vi "Polynom Daten speichern.vi"(6 "Aktionen":T3, 7 "Aktuelle Gasliste FT-IR":T1[](array[typedef]), 8 "Aktiv":bool[](array[boolean]), 9 "Polynome":dbl[][](array[numeric]) format="%#_18f", 10 "Einzelnes Polynom":dbl[](array[numeric]), 11 "Komponente":u16) -> (0 "Aktiv":bool[](array[boolean]), 1 "Polynome":dbl[][](array[numeric]) format="%#_18g", 2 "Namen":string[](array[string]), 3 "Polynome":T2 {"Polynom" format="%#_20f"}, 4 "Einzelnes Polynom out":dbl[](array[numeric]), 5 "einzelnes aktiv":bool)   [LabVIEW 2020, in "Linearisierung v2.lvlib"]
uses:
  Linearisierung v2.lvlib
  Aktionen Polynom Daten speichern.ctl
  Polynome.ctl
  Visualisierungs Elemente/String - Ausgabefeld.ctl
  Allgemein/allgemeine Sub-VIs.lvlib
  Seiten/Gaszuordnung AO/Gaszuordnung AO.lvlib
  Polynomkoeffizientenanzeige.ctl
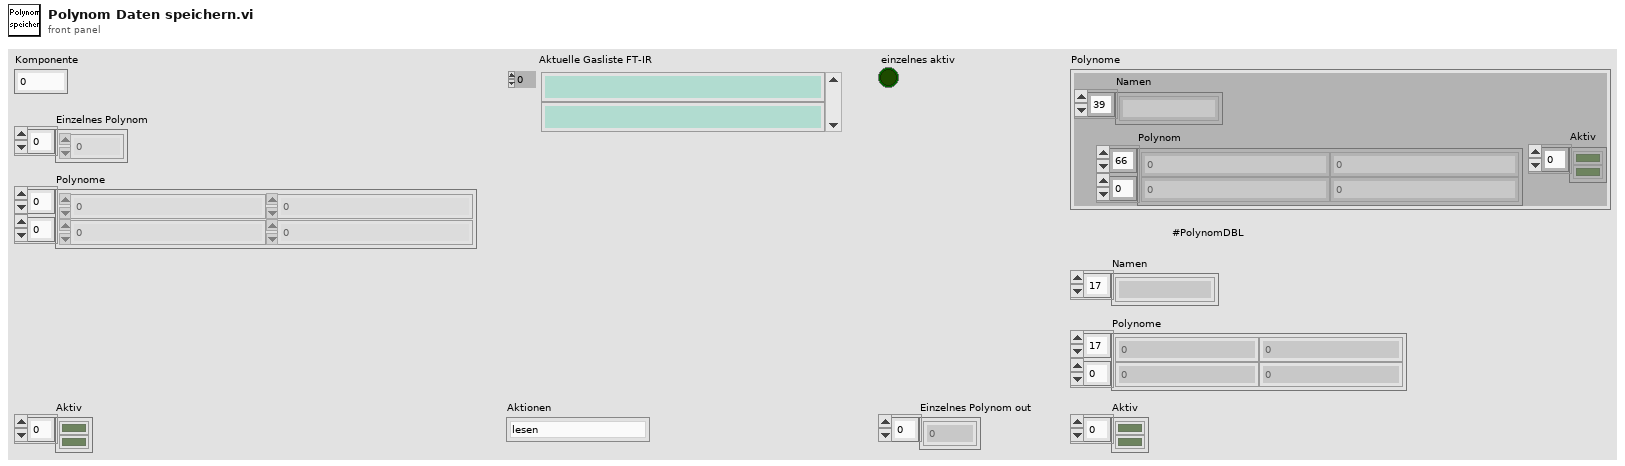
[diagram p1: front panel]
types:
  T1 = typedef "String - Ausgabefeld.ctl" = string
  T2 = typedef "Linearisierung v2.lvlib/Polynome.ctl" = cluster{"Namen":string[], "Polynom":dbl[][], "Aktiv":bool[]}
  T3 = typedef "Linearisierung v2.lvlib/Aktionen Polynom Daten speichern.ctl" = enum16{"lesen", "laden", "speichern", "schreiben", "schreiben alle", "Liste erstellen", "aktivieren", "deaktivieren", "aktiv abfragen"}
  T4 = enum16{"open", "replace", "create", "open or create", "replace or create", "replace or create with confirmation"}
  T5 = typedef "Linearisierung v2.lvlib/Polynomkoeffizientenanzeige.ctl" = cluster{"Offset":dbl, "O.1":dbl, "O. 2":dbl, "O. 3":dbl, "O. 4":dbl}
  T6 = cluster{"Namen":string[], "Polynom":dbl[][], "Aktiv":bool[]}
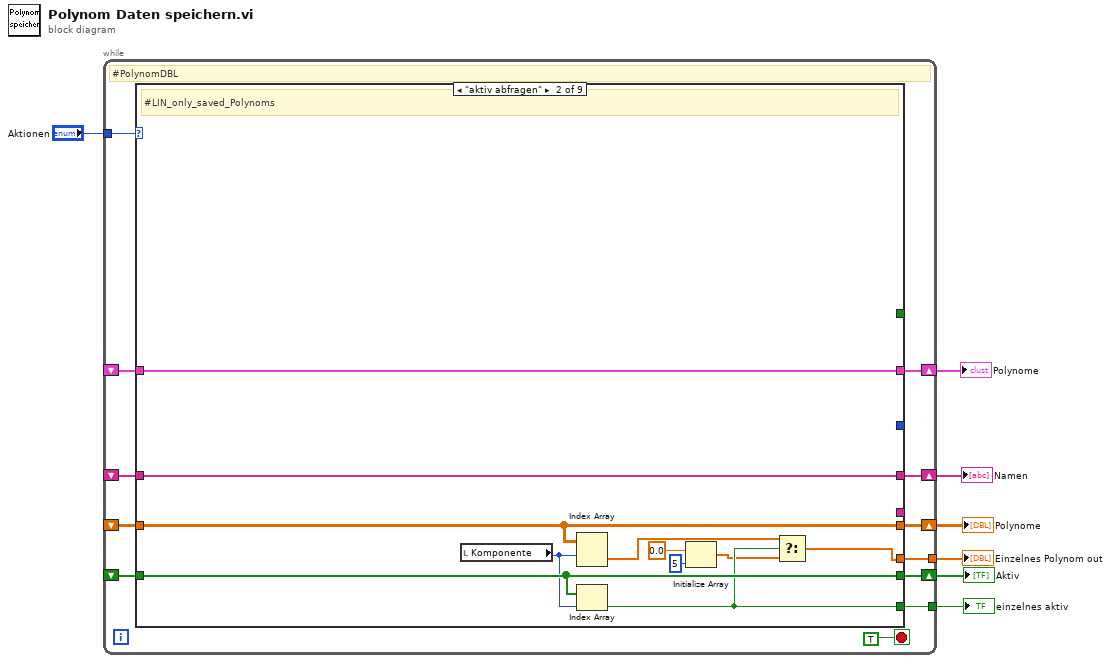
[diagram p0: block diagram]
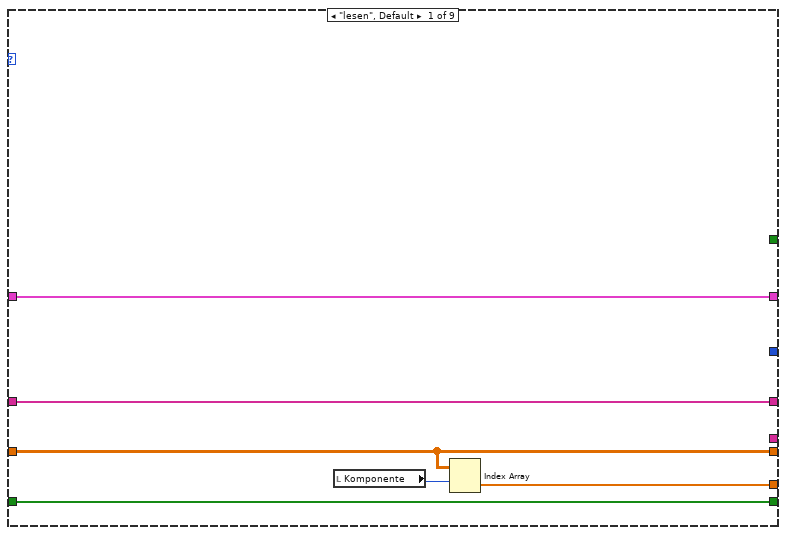
[diagram p2: hidden frame]
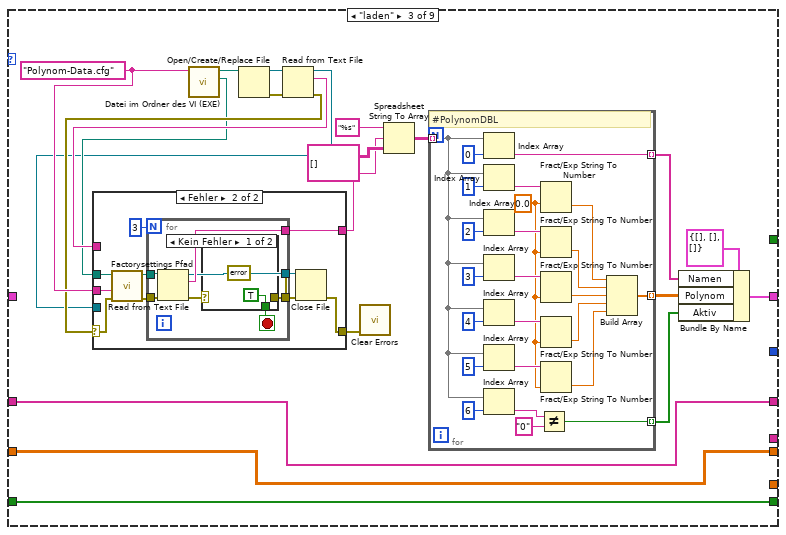
[diagram p3: hidden frame]
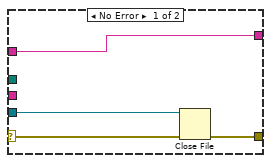
[diagram p4: hidden frame]
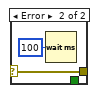
[diagram p5: hidden frame]
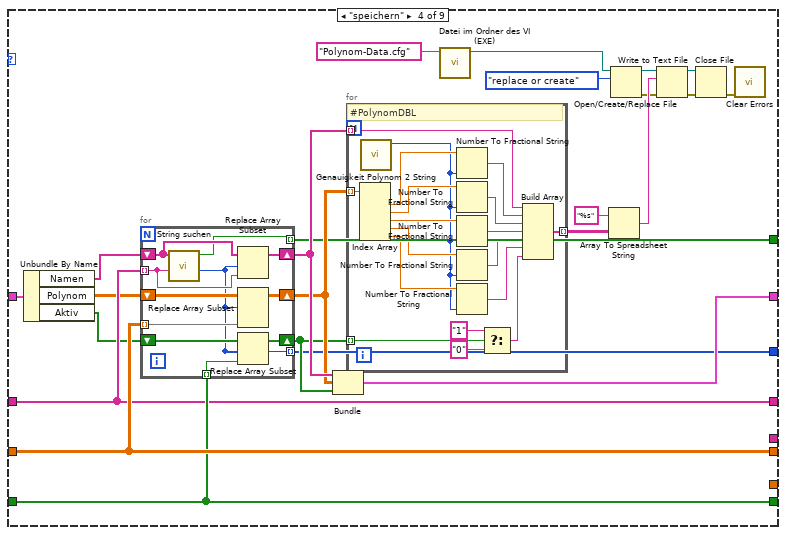
[diagram p6: hidden frame]
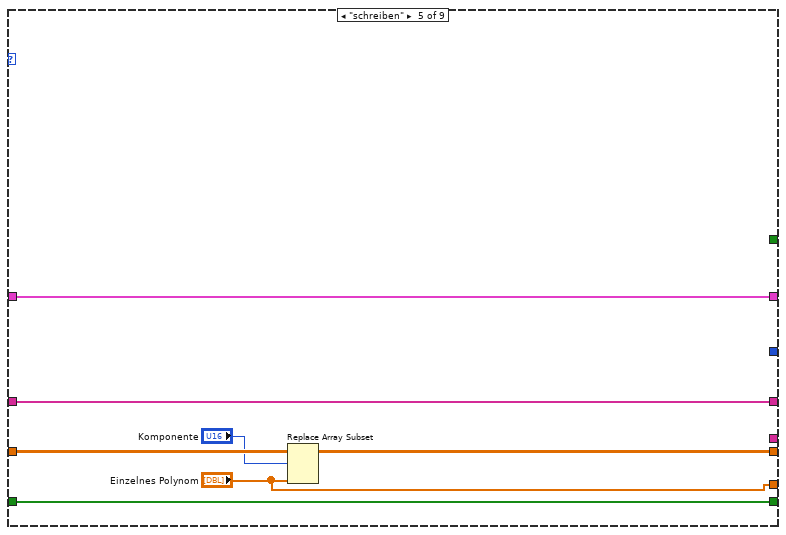
[diagram p7: hidden frame]
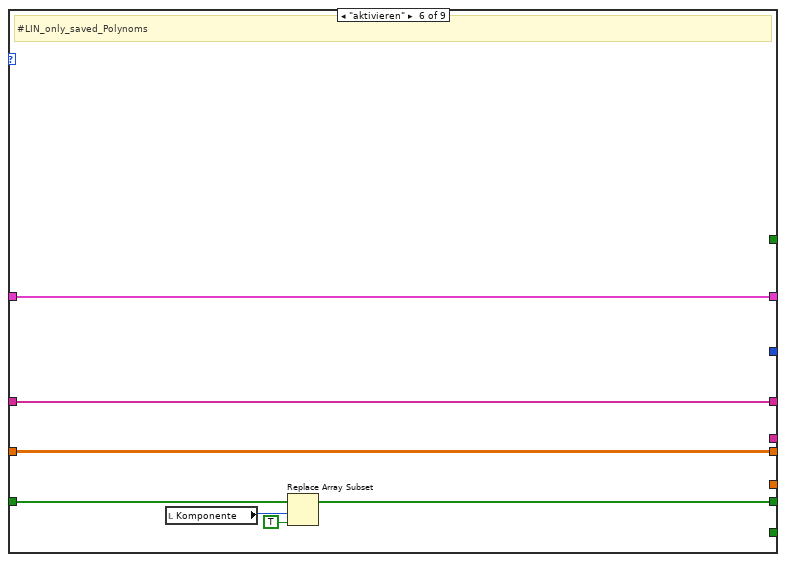
[diagram p8: hidden frame]
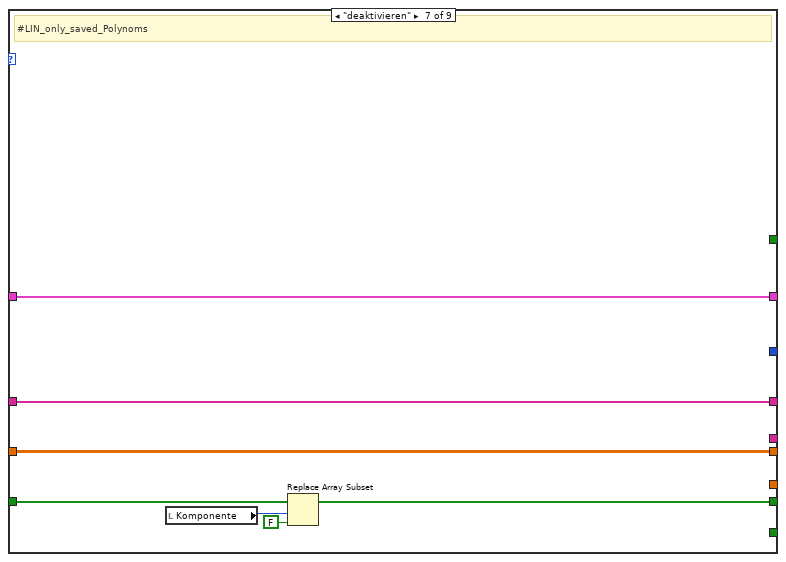
[diagram p9: hidden frame]
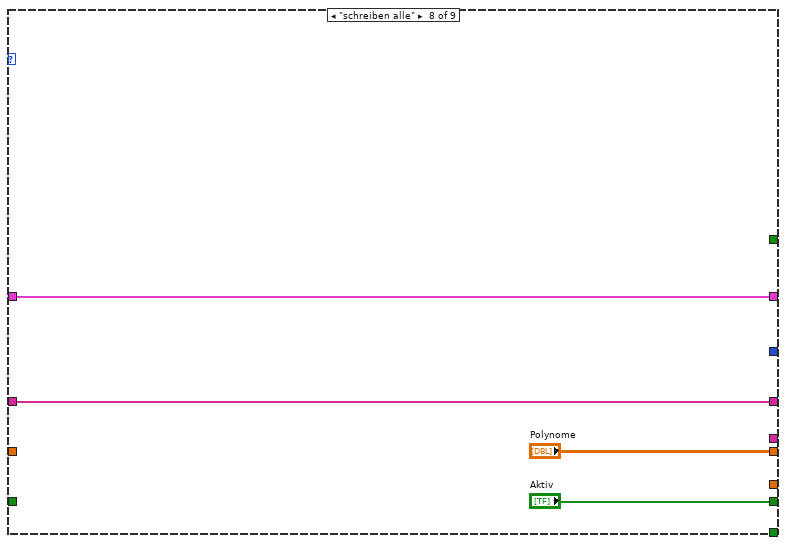
[diagram p10: hidden frame]
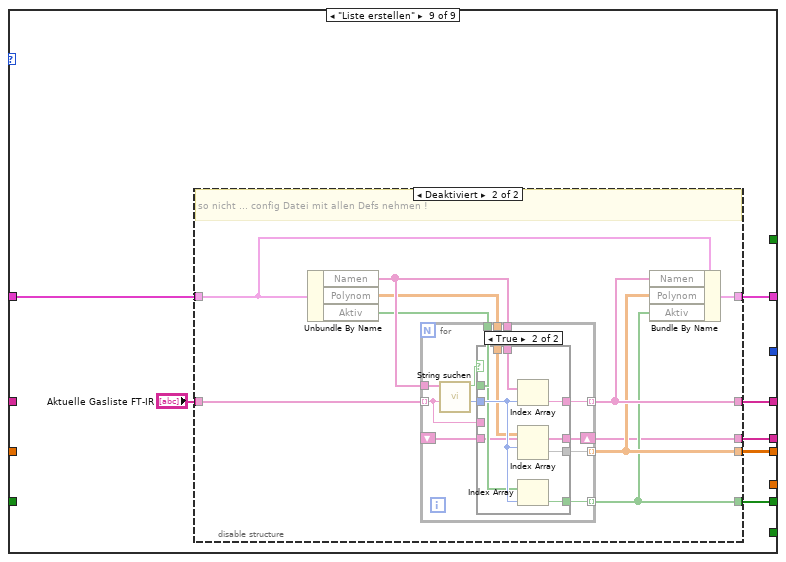
[diagram p11: hidden frame]
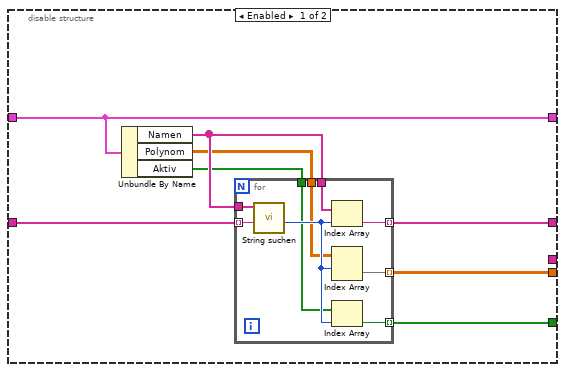
[diagram p12: hidden frame]
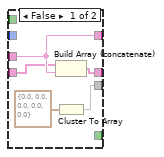
[diagram p13: hidden frame]
diagram:
  n1 = while {
    tunnel: "Aktionen" -> [w18]
    shift-right: [w17] -> w6
    shift-left: _ -> [w16]
    shift-right: [w13] -> w3
    shift-left: _ -> [w12]
    shift-right: [w14] -> w4
    shift-left: _ -> [w11]
    shift-right: [w15] -> w5
    shift-left: _ -> [w10]
    tunnel: [w9] -> w2
    tunnel: [w8] -> w1
    stop <- TRUE stop-if-true
    # "#PolynomDBL"
    n2 = case shown="\"aktiv abfragen\"" w18 {
      tunnel: [w25 w36 w44 w118 w163 w171 w178 w181 w187] -> w17
      tunnel: w16 -> [w25 w36 _ w120 w163 w171 w178 w181 w191]
      tunnel: [w23 w33 w47 w117 w161 w167 w174 "Aktiv" w190] -> w15
      tunnel: [w22 w34 w46 w119 w164 w172 w179 "Polynome" w189] -> w14
      tunnel: [w24 w35 w45 w112 w166 w173 w180 w184 w188] -> w13
      tunnel: w12 -> [w24 w35 w45 w112 w166 w173 w180 w184 _]
      tunnel: w11 -> [w22 w34 w46 w119 w165 w172 w179 _ _]
      tunnel: w10 -> [w23 w33 w47 w117 w161 w170 w177 _ _]
      tunnel: [w20 w29 _ _ "Einzelnes Polynom" _ _ _ _] -> w9
      tunnel: [_ _ _ w108 _ _ _ _ _] -> _
      tunnel: [_ _ _ _ _ _ _ _ w185] -> _
      tunnel: [_ _ _ w107 _ _ _ _ _] -> _
      tunnel: [_ w30 _ _ _ _ _ _ _] -> w8
      frame "lesen", Default {
        n3 = local read "Komponente"() -> (w21:u16)
        n4 = Index Array(array=w22, index (row)=w21) -> (element=w20:dbl[])  [unwired: 1 in]
      }
      frame "aktiv abfragen" {
        # "#LIN_only_saved_Polynoms"
        n5 = local read "Komponente"() -> (w32:u16)
        n6 = Index Array(array=w34, index (row)=w32) -> (element=w31:dbl[])  [unwired: 1 in]
        n7 = Index Array(array=w33, index=w32) -> (element=w30:bool)
        n8 = Initialize Array(0.0 ("Numerisch"), 5 ("Dimensionsgröße")) -> (w26:dbl[])
        n9 = Select(t=w31, s=w30, f=w26) -> (s? t:f=w29:dbl[])
      }
      frame "laden" {
        w40 = "Polynom-Data.cfg" ("Dateiname")
        n10 = call "Datei im Ordner des VI (EXE).vi"("Dateiname"=w40) -> ("Ordner des Haupt-VIs"=w38:path, "Dateipfad im Ordner des Haupt-VIs"=w52:path)  [unwired: 8 in, 1 out]
        n11 = Open/Create/Replace File(file path (use dialog)=w52) -> (refnum out=w54:refnum<file>, error out=w53:errorcluster)  [unwired: 1 in, 5 out]
        n12 = Read from Text File(file (use dialog)=w54, error in=w53) -> (refnum out=w37:refnum<file>, text=w41:string, error out=w39:errorcluster)  [unwired: 3 out]
        n13 = case shown="Fehler" w39 {
          selector: w39 -> [w60 w63]
          tunnel: w38 -> [_ w64]
          tunnel: w41 -> [w61 _]
          tunnel: [w61 w70] -> w42
          tunnel: [w58 w68] -> w43
          tunnel: w37 -> [w59 _]
          tunnel: w40 -> [_ w62]
          frame No Error {
            n14 = Close File(refnum=w59, error in=w60) -> (error out=w58:errorcluster)  [unwired: 1 out]
          }
          frame Error {
            n15 = call "Factorysettings Pfad.vi"("error in (no error)"=w63, "Dateiname"=w62, "Ordner des Haupt-VIs"=w64) -> ("error out"=w65:errorcluster, "Pfad Factorysettings"=w66:path)  [unwired: 7 in]
            n16 = for {
              N: 3 -> [_]
              tunnel: w65 -> [w76]
              tunnel: w66 -> [w75]
              tunnel: [w74] -> w70
              tunnel: [w73] -> w69
              tunnel: [w72] -> w67
              stop <- w77 stop-if-true
              n17 = Read from Text File(file (use dialog)=w75, error in=w76) -> (refnum out=w72:refnum<file>, text=w74:string, error out=w78:errorcluster)  [unwired: 2 in, 1 out]
              n18 = case shown="Kein Fehler" w78 {
                selector: w78 -> [_ w81]
                tunnel: [TRUE _] -> w77
                tunnel: [errorcluster {"status"=FALSE, "code"=0, "source"=""} ("error IO") w81] -> w73
                frame No Error {
                }
                frame Error {
                  n19 = Wait (ms)(milliseconds to wait=u32 100 ("Zu wartende ms")) -> ()  [unwired: 1 out]
                }
              }
            }
            n20 = Close File(refnum=w67, error in=w69) -> (error out=w68:errorcluster)  [unwired: 1 out]
          }
        }
        n21 = call <vilib>:"Clear Errors.vi"("error in (no error)"=w43) -> ()  [unwired: 5 in, 2 out]
        n22 = Spreadsheet String To Array(format string="%s" ("Format-String"), spreadsheet string=w42, array type (2D Dbl)=string[][] []) -> (array=w57:string[][])  [unwired: 1 out]
        n23 = for {
          tunnel: w57 -> [w93] mode=indexing
          tunnel: [w103] -> w48 mode=indexing
          tunnel: [w90] -> w50 mode=indexing
          tunnel: [w84] -> w49 mode=indexing
          w83 = 0.0 ("Standard (0 DBL)")
          # "#PolynomDBL"
          n24 = Index Array(array=w93, index=0 ("Index")) -> (element=w103:string)
          n25 = Index Array(array=w93, index=1 ("Index")) -> (element=w102:string)
          n26 = Index Array(array=w93, index=2 ("Index")) -> (element=w101:string)
          n27 = Index Array(array=w93, index=3 ("Index")) -> (element=w100:string)
          n28 = Index Array(array=w93, index=4 ("Index")) -> (element=w97:string)
          n29 = Index Array(array=w93, index=5 ("Index")) -> (element=w96:string)
          n30 = Index Array(array=w93, index=6 ("Index")) -> (element=w91:string)
          n31 = Not Equal?(x=w91, y="0") -> (x != y?=w90:bool)
          n32 = Fract/Exp String To Number(string=w102, default (0 dbl)=w83) -> (number=w89:dbl)  [unwired: 3 out]
          n33 = Fract/Exp String To Number(string=w101, default (0 dbl)=w83) -> (number=w88:dbl)  [unwired: 3 out]
          n34 = Fract/Exp String To Number(string=w100, default (0 dbl)=w83) -> (number=w87:dbl)  [unwired: 3 out]
          n35 = Fract/Exp String To Number(string=w97, default (0 dbl)=w83) -> (number=w86:dbl)  [unwired: 3 out]
          n36 = Fract/Exp String To Number(string=w96, default (0 dbl)=w83) -> (number=w85:dbl)  [unwired: 3 out]
          n37 = Build Array(w89, w88, w87, w86, w85) -> (w84:dbl[])
        }
        n38 = Bundle By Name(cluster=T2 {"Namen"=[], "Polynom"=[], "Aktiv"=[]} ("Polynome"), "Namen"=w48, "Polynom"=w49, "Aktiv"=w50) -> (w44:T2)
      }
      frame "speichern" {
        n39 = Unbundle By Name(w120) -> ("Namen"=w111:string[], "Polynom"=w109:dbl[][], "Aktiv"=w110:bool[])
        n40 = for {
          tunnel: w112 -> [w154] mode=indexing
          tunnel: w119 -> [w159] mode=indexing
          tunnel: w117 -> [w155] mode=indexing
          shift-right: [w158] -> w115
          shift-left: w111 -> [w153]
          shift-right: [w157] -> w114
          shift-left: w109 -> [w151]
          shift-right: [w156] -> w113
          shift-left: w110 -> [w152]
          tunnel: [w150] -> w108 mode=indexing
          tunnel: [w149] -> w107 mode=indexing
          n41 = call "String suchen.vi"("Gasname"=w154, "Such-Namen"=w153) -> ("Index"=w149:i32, "Gefunden?"=w150:bool)  [unwired: 8 in]
          n42 = Replace Array Subset(array=w153, new element=w154, index=w149) -> (w158:string[])
          n43 = Replace Array Subset(array=w151, new element=w159, index (row)=w149) -> (w157:dbl[][])  [unwired: 1 in]
          n44 = Replace Array Subset(array=w152, new element=w155, index=w149) -> (w156:bool[])
        }
        n45 = Bundle("Namen"=w115, "Polynom"=w114, "Aktiv"=w113) -> (w118:T6)  [unwired: 1 in]
        n46 = for {
          tunnel: w115 -> [w148] mode=indexing
          tunnel: [w145] -> w116 mode=indexing
          tunnel: w113 -> [w142] mode=indexing
          tunnel: w114 -> [w137] mode=indexing
          # "#PolynomDBL"
          n47 = Index Array(array=w137) -> (element #1=w136:dbl, element #2=w132:dbl, element #3=w133:dbl, element #4=w134:dbl, element #5=w135:dbl)  [unwired: 5 in]
          n48 = call "Genauigkeit Polynom 2 String.vi"() -> ("Genauigkeit Polynom 2 String"=w131:i16)  [unwired: 9 in, 2 out]
          n49 = Number To Fractional String(number=w136, precision (6)=w131) -> (F-format string=w147:string)  [unwired: 2 out]
          n50 = Number To Fractional String(number=w132, precision (6)=w131) -> (F-format string=w146:string)  [unwired: 2 out]
          n51 = Number To Fractional String(number=w133, precision (6)=w131) -> (F-format string=w141:string)  [unwired: 2 out]
          n52 = Number To Fractional String(number=w134, precision (6)=w131) -> (F-format string=w140:string)  [unwired: 2 out]
          n53 = Number To Fractional String(number=w135, precision (6)=w131) -> (F-format string=w139:string)  [unwired: 2 out]
          n54 = Select(t="1", s=w142, f="0") -> (s? t:f=w138:string)
          n55 = Build Array(w148, w147, w146, w141, w140, w139, w138) -> (w145:string[])
        }
        n56 = call "Datei im Ordner des VI (EXE).vi"("Dateiname"="Polynom-Data.cfg") -> ("Dateipfad im Ordner des Haupt-VIs"=w122:path)  [unwired: 8 in, 2 out]
        n57 = Array To Spreadsheet String(array=w116, 3:"%s" ("Format-String")) -> (spreadsheet string=w127:string)  [unwired: 1 out]
        n58 = Open/Create/Replace File(file path (use dialog)=w122, operation (0:open)=T4."replace or create" ("Operation (0:Öffnen)")) -> (refnum out=w128:refnum<file>, error out=w124:errorcluster)  [unwired: 1 in, 4 out]
        n59 = Write to Text File(file (use dialog)=w128, text=w127, error in=w124) -> (refnum out=w125:refnum<file>, error out=w126:errorcluster)  [unwired: 2 out]
        n60 = Close File(refnum=w125, error in=w126) -> (error out=w121:errorcluster)  [unwired: 1 out]
        n61 = call <vilib>:"Clear Errors.vi"("error in (no error)"=w121) -> ()  [unwired: 5 in, 2 out]
      }
      frame "schreiben" {
        n62 = Replace Array Subset(array=w165, new element="Einzelnes Polynom", index (row)="Komponente") -> (w164:dbl[][])  [unwired: 1 in]
      }
      frame "aktivieren" {
        # "#LIN_only_saved_Polynoms"
        n63 = local read "Komponente"() -> (w169:u16)
        n64 = Replace Array Subset(array=w170, new element=TRUE ("Neues Element/Teil-Array"), index=w169) -> (w167:bool[])
      }
      frame "deaktivieren" {
        # "#LIN_only_saved_Polynoms"
        n65 = local read "Komponente"() -> (w176:u16)
        n66 = Replace Array Subset(array=w177, new element=FALSE ("Neues Element/Teil-Array"), index=w176) -> (w174:bool[])
      }
      frame "schreiben alle" {
      }
      frame "Liste erstellen" {
        n67 = disable-structure shown="Deaktiviert" {
          disable-tunnel: w191 -> [w193 w215]
          disable-tunnel: [w196 w212] -> w190
          disable-tunnel: [w195 w213] -> w189
          disable-tunnel: [w194 w214] -> w188
          disable-tunnel: [w193 w211] -> w187
          disable-tunnel: "Aktuelle Gasliste FT-IR" -> [w192 w210]
          disable-tunnel: [_ w209] -> w185
          frame Enabled {
            n68 = Unbundle By Name(w193) -> ("Namen"=w199:string[], "Polynom"=w198:dbl[][], "Aktiv"=w197:bool[])
            n69 = for {
              tunnel: w192 -> [w208] mode=indexing
              tunnel: w199 -> [w207]
              tunnel: w199 -> [w205]
              tunnel: w198 -> [w204]
              tunnel: w197 -> [w203]
              tunnel: [w202] -> w194 mode=indexing
              tunnel: [w201] -> w195 mode=indexing
              tunnel: [w200] -> w196 mode=indexing
              n70 = call "String suchen.vi"("Gasname"=w208, "Such-Namen"=w207) -> ("Index"=w206:i32)  [unwired: 8 in, 1 out]
              n71 = Index Array(array=w205, index=w206) -> (element=w202:string)
              n72 = Index Array(array=w204, index (row)=w206) -> (element=w201:dbl[])  [unwired: 1 in]
              n73 = Index Array(array=w203, index=w206) -> (element=w200:bool)
            }
          }
          frame Disabled {
            # "so nicht ... config Datei mit allen Defs nehmen !"
            n74 = Unbundle By Name(w215) -> ("Namen"=w218:string[], "Polynom"=w217:dbl[][], "Aktiv"=w216:bool[])
            n75 = for {
              tunnel: w210 -> [w221] mode=indexing
              tunnel: w218 -> [w230]
              tunnel: w218 -> [w228]
              tunnel: w217 -> [w227]
              tunnel: w216 -> [w226]
              tunnel: [w225] -> w214 mode=indexing
              tunnel: [w224] -> w213 mode=indexing
              tunnel: [w223] -> w212 mode=indexing
              shift-right: [w220] -> w209
              shift-left: _ -> [w219]
              n76 = call "String suchen.vi"("Gasname"=w221, "Such-Namen"=w230) -> ("Index"=w229:i32, "Gefunden?"=w222:bool)  [unwired: 8 in]
              n77 = case shown="True" w222 {
                tunnel: w229 -> [_ w243]
                tunnel: w228 -> [_ w242]
                tunnel: w227 -> [_ w241]
                tunnel: w226 -> [_ w240]
                tunnel: [w235 w239] -> w225
                tunnel: [w231 w238] -> w224
                tunnel: [_ w237] -> w223
                tunnel: w221 -> [w235 _]
                tunnel: [w234 w236] -> w220
                tunnel: w219 -> [w233 w236]
                frame False {
                  n78 = Build Array (concatenate)(w233, w235) -> (w234:T1[])
                  n79 = Cluster To Array(cluster=T5 {"Offset"=0.0, "O.1"=0.0, "O. 2"=0.0, "O. 3"=0.0, "O. 4"=0.0} ("Polynomkoeffizienten")) -> (array=w231:dbl[])
                }
                frame True {
                  n80 = Index Array(array=w242, index=w243) -> (element=w239:string)
                  n81 = Index Array(array=w241, index (row)=w243) -> (element=w238:dbl[])  [unwired: 1 in]
                  n82 = Index Array(array=w240, index=w243) -> (element=w237:bool)
                }
              }
            }
            n83 = Bundle By Name(cluster=w215, "Namen"=w214, "Polynom"=w213, "Aktiv"=w212) -> (w211:T2)
          }
        }
      }
    }
  }
  "Polynome" <- w6
  "Aktiv" <- w5
  "Polynome" <- w4
  "Namen" <- w3
  "Einzelnes Polynom out" <- w2
  "einzelnes aktiv" <- w1
